vi "XIPIN_AXI4-Stream_Register_Slice_1_1.vi"   [LabVIEW 2017]
doc: "The AXI4-Stream Register Slice IP provides the infrastructure to insert a pipeline stage between a AXI4-Stream master and slave.\n------------------------------------\n<b>Need License</b> : No\n<b>Interface</b> : AXI4-Stream"
uses:
  <vilib>/rvi/XilinxIP/XIPIN_XNode/niFpgaXIPIN.xnode
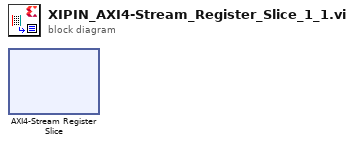
[diagram p0: block diagram]
diagram:
  n1 = xnode ("AXI4-Stream Register Slice")() -> ()
